vi "Stop Core.vi"(10 "final error code":i32, 11 "Tcp in":refnum<class "Tcp.lvclass">) -> (3 "Tcp out":refnum<class "Tcp.lvclass">)   [LabVIEW 2022 SP3, in "Tcp.lvlib" / "Tcp.lvclass"]
doc: "(<B>Filename</B>: Actor Framework.lvlib:Actor.lvclass:Stop Core.vi)\n\nDefines what the actor does before it stops. Use the <B>final error code</B> input to determine whether the actor shut down in response to an error.\n\nBy default, this method does nothing. A descendant class may override it to define behavior, such as shutting down any processes the actor initiated in its override of the Actor Core method."
uses:
  Tcp.lvclass
  <vilib>/ActorFramework/Actor/Actor.lvclass
  TcpSocket/Source/TcpSocket/TcpServer/TcpServer.lvclass
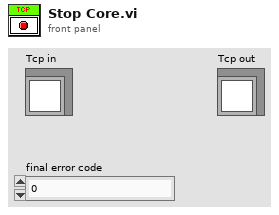
[diagram p1: front panel]
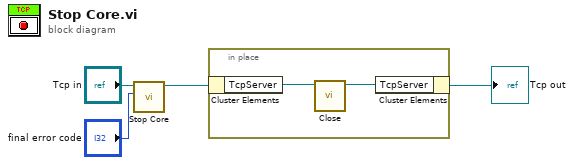
[diagram p0: block diagram]
diagram:
  n1 = call-parent "Stop Core.vi"("final error code"="final error code", "Actor in"="Tcp in") -> ("Actor out"=w2:refnum<class "Tcp.lvclass">)  [unwired: 9 in]
  n2 = in-place {
    n3 = in-place-cluster #1(w2) -> ("TcpServer"=w6:refnum<class "TcpServer.lvclass">)
    n4 = call-dynamic "Close.vi"("TcpSocket in"=w6) -> ("TcpSocket out"=w5:refnum<class "TcpServer.lvclass">)  [unwired: 9 in, 1 out]
    n5 = in-place-cluster #1("TcpServer"=w5) -> (→"Tcp out":refnum<class "Tcp.lvclass">)
  }
